vi "Instrument Command Response.vi"(8 "error in (no error)":errorcluster, 10 "Command Parameters":T2, 11 "Comm.Info":T4) -> (0 "error out":errorcluster, 1 "Timed Out?":bool, 2 "Response":T1, 3 "Comm.Info":T4)   [LabVIEW 2020, in "Instrument Host Automation API.lvlib"]
uses:
  Instrument Host Automation API.lvlib
  <vilib>/NI/STM/TCP/TCP Connection Info.ctl
  <vilib>/NI/STM/SubVIs/MetaDataElement.ctl
  Addon/Addon Shared/Types/Buffered RT Instrument Command.ctl
  Addon/Addon Shared/Types/Response Wait Type.ctl
  Addon/Addon Shared/Types/Buffered RT Instrument Request.ctl
  Addon/Addon Shared/Instrument Addon Shared.lvlib
  <vilib>/NI/NI VeriStand Addon Network Comm/Shared/NI VeriStand Addon Network Comm Shared.lvlib
  <vilib>/NI/STM/NI STM.lvlib
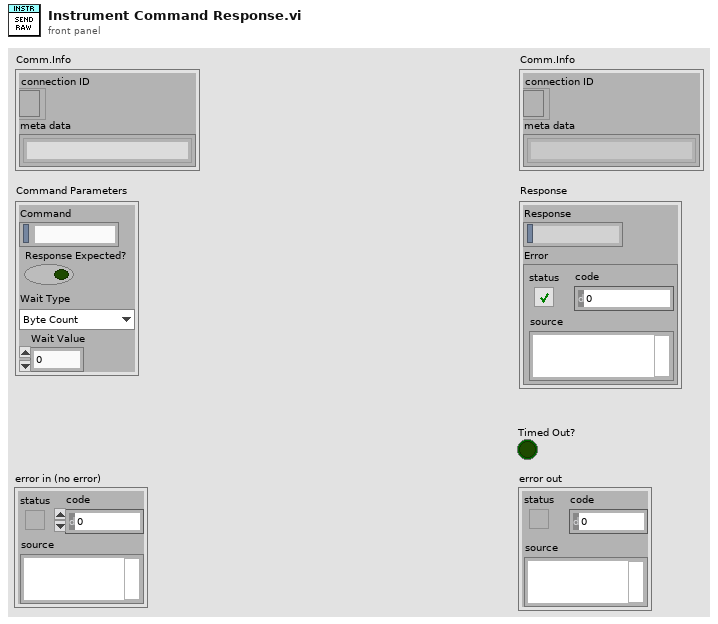
[diagram p1: front panel]
types:
  T1 = typedef "Instrument Addon Shared.lvlib/Buffered RT Instrument Request.ctl" = cluster{"Response":string, "Error":errorcluster}
  T2 = typedef "Instrument Addon Shared.lvlib/Buffered RT Instrument Command.ctl" = cluster{"Command":string, "Response Expected?":bool, "Wait Type":T3, "Wait Value":dbl}
  T3 = typedef "Instrument Addon Shared.lvlib/Response Wait Type.ctl" = enum16{"Byte Count", "Wait sec"}
  T4 = typedef "NI STM.lvlib/TCP Connection Info.ctl" = cluster{"connection ID":refnum<k5>, "meta data":T5[]}
  T5 = typedef "NI STM.lvlib/MetaDataElement.ctl" = string
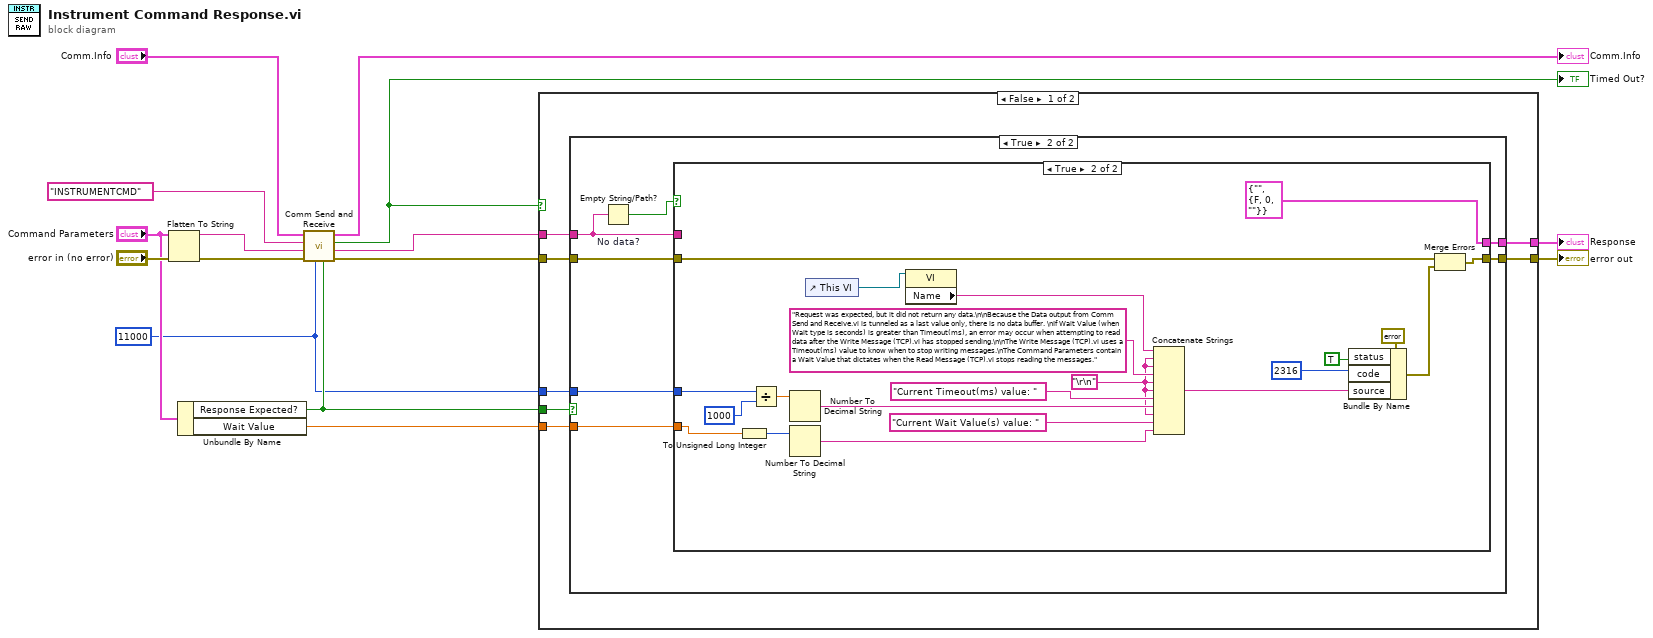
[diagram p0: block diagram]
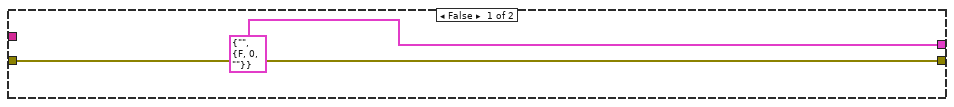
[diagram p2: hidden frame]
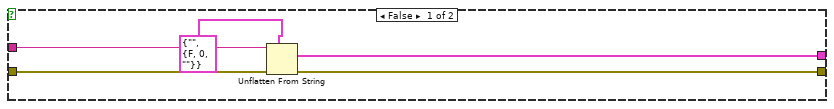
[diagram p3: hidden frame]
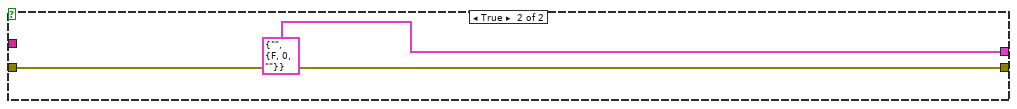
[diagram p4: hidden frame]
diagram:
  w2 = u32 11000 ("Timeout (ms)")
  n1 = Flatten To String(anything="Command Parameters", error in (no error)="error in (no error)") -> (data string=w6:string, error out=w11:errorcluster)  [unwired: 2 in, 1 out]
  n2 = Unbundle By Name("Command Parameters") -> ("Response Expected?"=w3:bool, "Wait Value"=w1:dbl)
  n3 = call <vilib>:"Comm Send and Receive.vi"("Resp Required?"=w3, "Timeout (ms)"=w2, "error in (no error)"=w11, "Data"=w6, "Name"="INSTRUMENTCMD", "connection info"="Comm.Info") -> ("error out"=w9:errorcluster, "Data"=w10:string, "Timed Out?"=w5:bool, "connection info"=→"Comm.Info":T4)  [unwired: 2 in]
  "Timed Out?" <- w5
  n4 = case shown="False" w5 {
    tunnel: w10 -> [w22 _]
    tunnel: w9 -> [w21 w59]
    tunnel: [w20 w59] -> w8
    tunnel: [w19 T1 {"Response"="", "Error"={"status"=FALSE, "code"=0, "source"=""}} ("Cluster")] -> w7
    tunnel: w3 -> [w18 _]
    tunnel: w2 -> [w17 _]
    tunnel: w1 -> [w16 _]
    frame False {
      n5 = case shown="True" w18 {
        tunnel: w22 -> [_ w27]
        tunnel: w21 -> [w23 w31]
        tunnel: [w23 w30] -> w20
        tunnel: [T1 {"Response"="", "Error"={"status"=FALSE, "code"=0, "source"=""}} ("Cluster") w29] -> w19
        tunnel: w17 -> [_ w26]
        tunnel: w16 -> [_ w25]
        frame False {
        }
        frame True {
          n6 = Empty String/Path? "No data?"(string/path=w27) -> (empty?=w28:bool)
          n7 = case shown="True" w28 {
            tunnel: w27 -> [w36 _]
            tunnel: w31 -> [w35 w55]
            tunnel: [w34 w56] -> w30
            tunnel: [w32 T1 {"Response"="", "Error"={"status"=FALSE, "code"=0, "source"=""}} ("Cluster")] -> w29
            tunnel: w26 -> [_ w38]
            tunnel: w25 -> [_ w39]
            frame False {
              n8 = Unflatten From String(type=T1 {"Response"="", "Error"={"status"=FALSE, "code"=0, "source"=""}} ("Cluster"), binary string=w36, error in (no error)=w35) -> (value=w32:T1, error out=w34:errorcluster)  [unwired: 2 in, 1 out]
            }
            frame True {
              w40 = "\r\n"
              n9 = To Unsigned Long Integer(number=w39) -> (unsigned 32bit integer=w49:u32)
              n10 = Divide(x=w38, y=u32 1000) -> (x/y=w47:dbl)
              n11 = Number To Decimal String(number=w47) -> (decimal integer string=w53:string)  [unwired: 1 in]
              n12 = Number To Decimal String(number=w49) -> (decimal integer string=w51:string)  [unwired: 1 in]
              n13 = control-ref of="This VI"() -> (w42:refnum<vi>)
              n14 = property class="VI"(reference=w42) -> ("Name"=w41:string)  [unwired: 1 in, 2 out]
              n15 = Concatenate Strings(w41, w40, w40, "Request was expected, but it did not return any data.\n\nBecause the Data output from Comm Send and Receive.vi is tunneled as a last value only, there is no data buffer. \nIf Wait Value (when Wait type is seconds) is greater than Timeout(ms), an error may occur when attempting to read data after the Write Message (TCP).vi has stopped sending.\n\nThe Write Message (TCP).vi uses a Timeout(ms) value to know when to stop writing messages.\nThe Command Parameters contain a Wait Value that dictates when the Read Message (TCP).vi stops reading the messages.", w40, w40, "Current Timeout(ms) value: ", w53, w40, "Current Wait Value(s) value: ", w51) -> (w43:string)
              n16 = Bundle By Name(cluster=errorcluster {"status"=FALSE, "code"=0, "source"=""} ("error in (no error)"), "status"=TRUE, "code"=2316 ("error code (0)"), "source"=w43) -> (w37:errorcluster)
              n17 = Merge Errors(w55, w37) -> (w56:errorcluster)
            }
          }
        }
      }
    }
    frame True {
    }
  }
  "error out" <- w8
  "Response" <- w7
